vi "VG_DeltaVcell.vi"() -> ()   [LabVIEW 2020]
panel:
  out "DeltaVcell":dbl
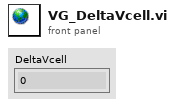
[diagram p1: front panel]
diagram:
